vi "Data string to info.vi"(8 "error in (no error)":errorcluster, 9 "Motor info":T2={"Motor positions"=[0.0, 0.0], "End-stop state"=[FALSE, FALSE], "°/step"=[], "Movement config"={"Direction motor 1"=1, "Direction motor 2"=1, "Step style motor 1"=1, "Step style motor 2"=1}} {"Movement config"."Step style motor 2" items=["", "Single", "Double", "Interleave", "Microstep"]; "Movement config"."Step style motor 1" items=["", "Single", "Double", "Interleave", "Microstep"]; "Movement config"."Direction motor 2" items=["", "Forward", "Backward"]; "Movement config"."Direction motor 1" items=["", "Initialize", "Move"]; "°/step" format="%#_13g"}, 10 "string":string) -> (0 "error out":errorcluster, 3 "Info out":T1)   [LabVIEW 2020, in "Arduino-Adafruit stepper.lvlib"]
uses:
  Arduino-Adafruit stepper.lvlib
  Motor info -- typedef.ctl
  Movement config -- typedef.ctl
  Motor direction.ctl
  Step style.ctl
  State info -- typedef.ctl
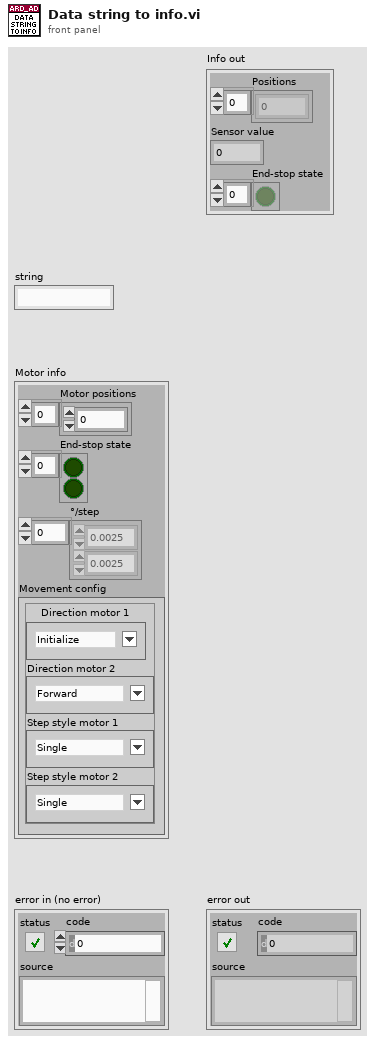
[diagram p1: front panel]
types:
  T1 = typedef "Arduino-Adafruit stepper.lvlib/State info -- typedef.ctl" = cluster{"Positions":dbl[], "Sensor value":dbl, "End-stop state":bool[]}
  T2 = typedef "Arduino-Adafruit stepper.lvlib/Motor info -- typedef.ctl" = cluster{"Motor positions":dbl[], "End-stop state":bool[], "°/step":dbl[], "Movement config":T3}
  T3 = typedef "Arduino-Adafruit stepper.lvlib/Movement config -- typedef.ctl" = cluster{"Direction motor 1":T4, "Direction motor 2":T4, "Step style motor 1":T5, "Step style motor 2":T5}
  T4 = typedef "Arduino-Adafruit stepper.lvlib/Motor direction.ctl" = u8
  T5 = typedef "Arduino-Adafruit stepper.lvlib/Step style.ctl" = u8
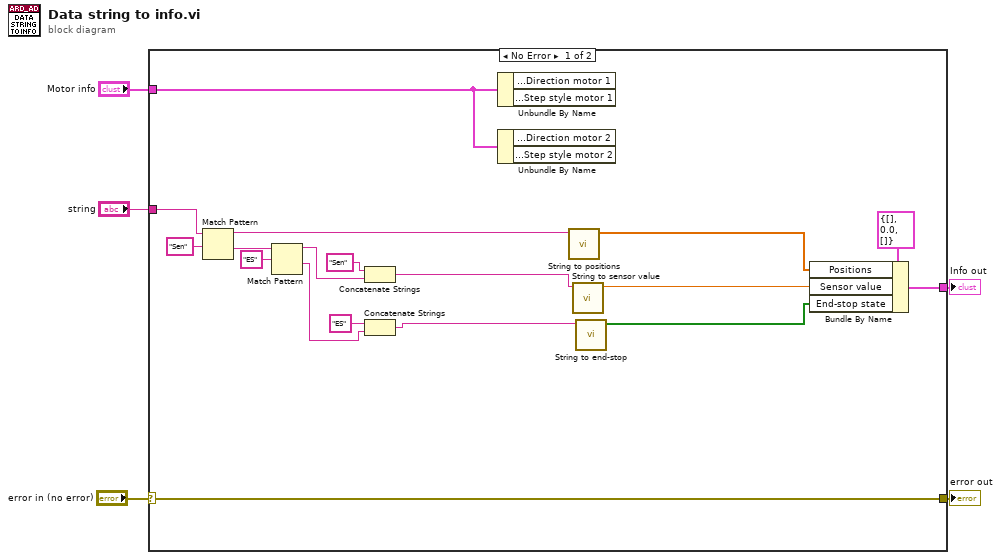
[diagram p0: block diagram]
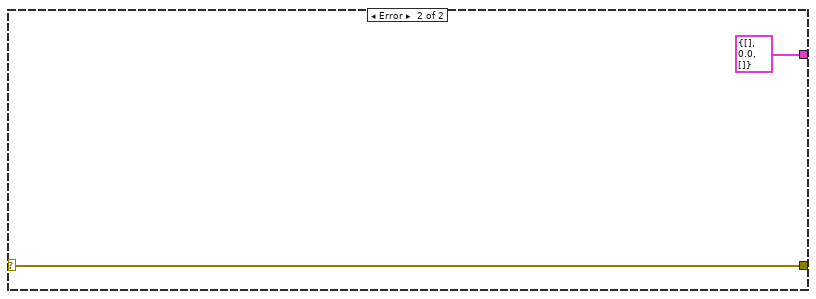
[diagram p2: hidden frame]
diagram:
  n1 = case shown="No Error" "error in (no error)" {
    selector: "error in (no error)" -> [w7 w24]
    tunnel: "Motor info" -> [w16 _]
    tunnel: "string" -> [w15 _]
    tunnel: [w8 T1 {"Positions"=[], "Sensor value"=0.0, "End-stop state"=[]} ("Info out")] -> w3
    tunnel: [w7 w24] -> w1
    frame No Error {
      n2 = Match Pattern(string=w15, regular expression="Sen") -> (before substring=w6:string, after substring=w19:string)  [unwired: 1 in, 2 out]
      n3 = Match Pattern(string=w19, regular expression="ES") -> (before substring=w18:string, after substring=w17:string)  [unwired: 1 in, 2 out]
      n4 = Concatenate Strings("Sen" ("string"), w18) -> (w14:string)
      n5 = Concatenate Strings("ES" ("string"), w17) -> (w13:string)
      n6 = Unbundle By Name(w16) -> ()  [unwired: 2 out]
      n7 = Unbundle By Name(w16) -> ()  [unwired: 2 out]
      n8 = call "String to positions.vi"("string"=w6) -> ("Array"=w11:dbl[])  [unwired: 9 in, 1 out]
      n9 = call "String to sensor value.vi"("String"=w14) -> ("Numeric"=w10:dbl)  [unwired: 10 in]
      n10 = call "String to end-stop.vi"("String"=w13) -> ("End-stop status"=w9:bool[])  [unwired: 9 in, 1 out]
      n11 = Bundle By Name(cluster=T1 {"Positions"=[], "Sensor value"=0.0, "End-stop state"=[]} ("Info out"), "Positions"=w11, "Sensor value"=w10, "End-stop state"=w9) -> (w8:T1)
    }
    frame Error {
    }
  }
  "error out" <- w1
  "Info out" <- w3
